vi "Log Hours to Array.vi"(6 "Display Array":string[](array[string]), 7 "Name doesn't exist?":bool, 8 "base path":path, 9 "Name Index":i32, 10 "Name":string, 11 "Display in":T1) -> (3 "Display out":T1)   [LabVIEW 2015]
uses:
  controls/Display Default.ctl
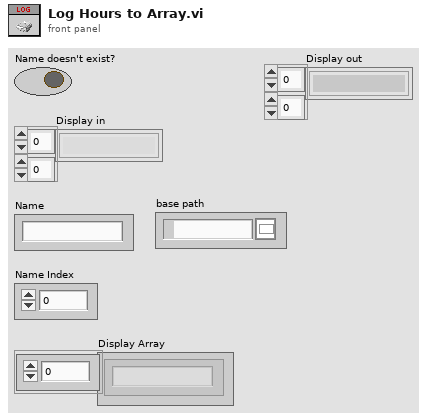
[diagram p1: front panel]
types:
  T1 = typedef "Display Default.ctl" = string[][]
  T2 = enum16{"open", "replace", "create", "open or create", "replace or create", "replace or create with confirmation"}
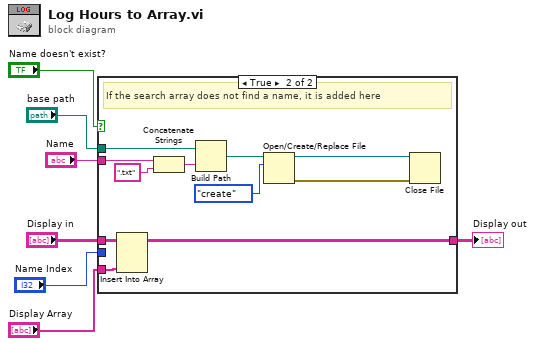
[diagram p0: block diagram]
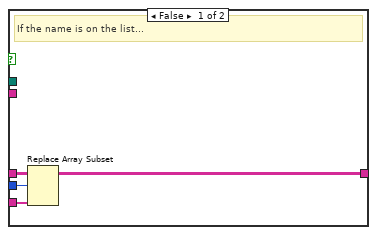
[diagram p2: hidden frame]
diagram:
  n1 = case shown="True" "Name doesn't exist?" {
    tunnel: "Display in" -> [w11 w22]
    tunnel: [w9 w20] -> w3
    tunnel: "Display Array" -> [w10 w21]
    tunnel: "Name Index" -> [w8 _]
    tunnel: "Name" -> [_ w13]
    tunnel: "base path" -> [_ w12]
    frame False {
      # "If the name is on the list..."
      n2 = Replace Array Subset(array=w11, new element=w10, index (row)=w8) -> (w9:T1)  [unwired: 1 in]
    }
    frame True {
      # "If the search array does not find a name, it is added here"
      n3 = Insert Into Array "Insert Into Array"(array=w22, new element=w21) -> (w20:T1)  [unwired: 2 in]
      n4 = Concatenate Strings(w13, ".txt" ("string")) -> (w19:string)
      n5 = Build Path(base path=w12, name or relative path=w19) -> (appended path=w18:path)
      n6 = Open/Create/Replace File(file path (use dialog)=w18, operation (0:open)=T2."create") -> (refnum out=w16:refnum<file>, error out=w15:errorcluster)  [unwired: 4 in, 1 out]
      n7 = Close File(refnum=w16, error in=w15) -> ()  [unwired: 2 out]
    }
  }
  "Display out" <- w3
